vi "GetGlobalDefaultConfiguration.vi"(2 "DO NOT override instruments":bool, 3 "Read defaults?":bool) -> (1 "Configuration File IV":path)   [LabVIEW 2013]
uses:
  QC_MeasurementSetup.vi
  InstrControl/InstrControl.lvclass
panel:
  out "Configuration File Cis":path
  out "Configuration File Stability":path
  out "Configuration File CV":path
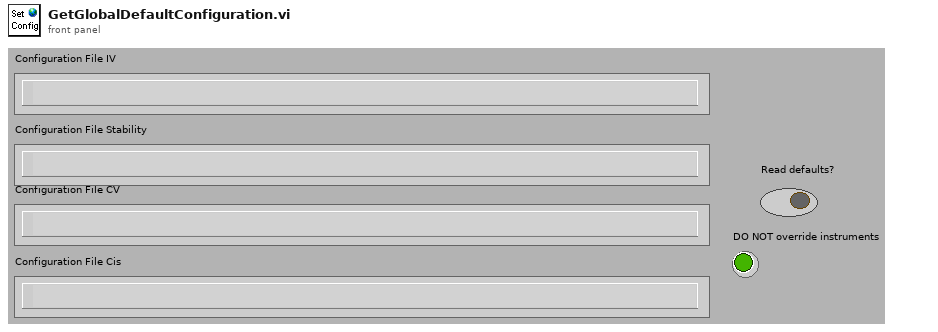
[diagram p1: front panel]
types:
  T1 = cluster{"Supply":refnum<class "SupplyControl.lvclass">, "Initial Voltage [V]":dbl, "Final Voltage [V]":dbl, "Step Size [V]":dbl, "Step Interval [s]":i32, "Number Of Steps":u32, "Ramp down steps [V]":dbl, "Ramp down Interval [s]":i32, "Set Current Limit?":bool, "Current Limit [µA]":dbl, "Temperature Readout":enum16{"Read Arduino", "Enter manually"}, "Arduino":refnum<class "ArduinoControl.lvclass">, "Supply Name":string, "V_breakdown Limit [V]":dbl, "Switching":refnum<class "Switching.lvclass">, "Matrix used?":bool, "Matrix X Channels":cluster{"Bias Supply / SMU LO":i32, "Bias Supply / SMU HI":i32, "CV Box LO":i32, "CV Box HI":i32, "CV Box LO IN":i32, "CV Box HI IN":i32, "Volt meter LO":i32, "Volt meter HI":i32, "Mux1 C1":i32, "Mux1 C2":i32, "Mux2 C1":i32, "Mux2 C2":i32}}
  T2 = cluster{"Supply":refnum<class "SupplyControl.lvclass">, "LCR":refnum<class "LCRControl.lvclass">, "Initial Voltage [V]":dbl, "Final Voltage [V]":dbl, "Step Size [V]":dbl, "Step Interval [s]":i32, "Number Of Steps":u32, "AC frequency [Hz]":i32, "RC Configuration":u16, "AC amplitude [V]":dbl, "Ramp down steps [V]":dbl, "Ramp down Interval [s]":i32, "Set Current Limit?":bool, "Current Limit [µA]":dbl, "Temperature Readout":enum16{"Read Arduino", "Enter manually"}, "Arduino":refnum<class "ArduinoControl.lvclass">, "Supply Name":string, "LCR Name":string, "V_depletion Limit [V]":dbl, "Switching":refnum<class "Switching.lvclass">, "Matrix used?":bool, "Matrix X Channels":cluster{"Bias Supply / SMU LO":i32, "Bias Supply / SMU HI":i32, "CV Box LO":i32, "CV Box HI":i32, "CV Box LO IN":i32, "CV Box HI IN":i32, "Volt meter LO":i32, "Volt meter HI":i32, "Mux1 C1":i32, "Mux1 C2":i32, "Mux2 C1":i32, "Mux2 C2":i32}}
  T3 = cluster{"Supply":refnum<class "SupplyControl.lvclass">, "Voltage [V]":dbl, "Measurement Interval [s]":i32, "Test Duration":u32, "Ramp up steps [V]":dbl, "Ramp up Interval [s]":u32, "Ramp down steps [V]":dbl, "Ramp down Interval [s]":i32, "Set Current Limit?":bool, "Current Limit [µA]":dbl, "Temperature Readout":enum16{"Read Arduino", "Enter manually"}, "Arduino":refnum<class "ArduinoControl.lvclass">, "Supply Name":string, "Maximum current fluctuation [%]":dbl, "Switching.lvclass":refnum<class "Switching.lvclass">, "Matrix used?":bool, "Matrix X Channels":cluster{"Bias Supply / SMU LO":i32, "Bias Supply / SMU HI":i32, "CV Box LO":i32, "CV Box HI":i32, "CV Box LO IN":i32, "CV Box HI IN":i32, "Volt meter LO":i32, "Volt meter HI":i32, "Mux1 C1":i32, "Mux1 C2":i32, "Mux2 C1":i32, "Mux2 C2":i32}}
  T4 = cluster{"Supply":refnum<class "SupplyControl.lvclass">, "LCR":refnum<class "LCRControl.lvclass">, "Initial Voltage [V]":dbl, "Final Voltage [V]":dbl, "Step Size [V]":dbl, "Step Interval [s]":i32, "Number Of Steps":u32, "AC frequency [Hz]":i32, "RC Configuration":u16, "AC amplitude [V]":dbl, "Ramp down steps [V]":dbl, "Ramp down Interval [s]":i32, "Set Current Limit?":bool, "Current Limit [µA]":dbl, "Temperature Readout":enum16{"Read Arduino", "Enter manually"}, "Arduino":refnum<class "ArduinoControl.lvclass">, "Supply Name":string, "LCR Name":string, "C_is Limit [pF/cm]":dbl, "Switching":refnum<class "Switching.lvclass">, "Matrix used?":bool, "Matrix X Channels":cluster{"Bias Supply / SMU LO":i32, "Bias Supply / SMU HI":i32, "CV Box LO":i32, "CV Box HI":i32, "CV Box LO IN":i32, "CV Box HI IN":i32, "Volt meter LO":i32, "Volt meter HI":i32, "Mux1 C1":i32, "Mux1 C2":i32, "Mux2 C1":i32, "Mux2 C2":i32}}
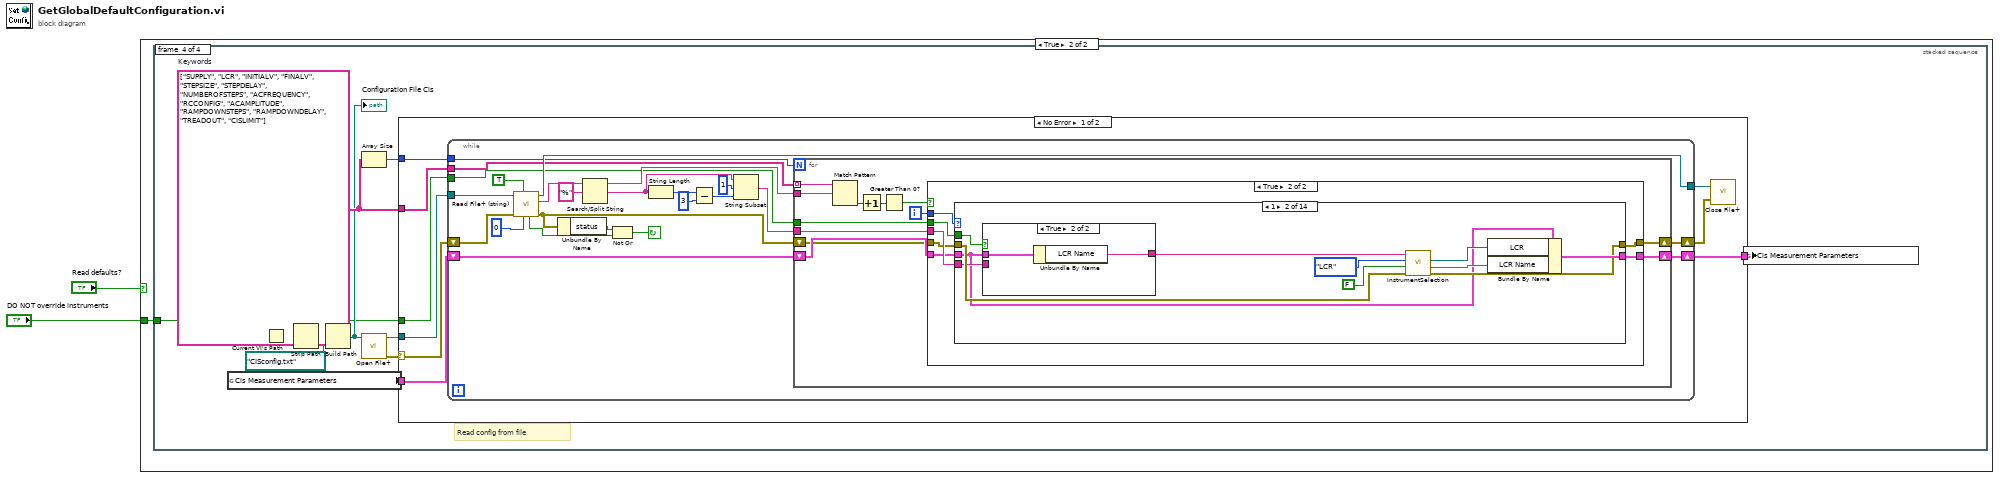
[diagram p0: block diagram]
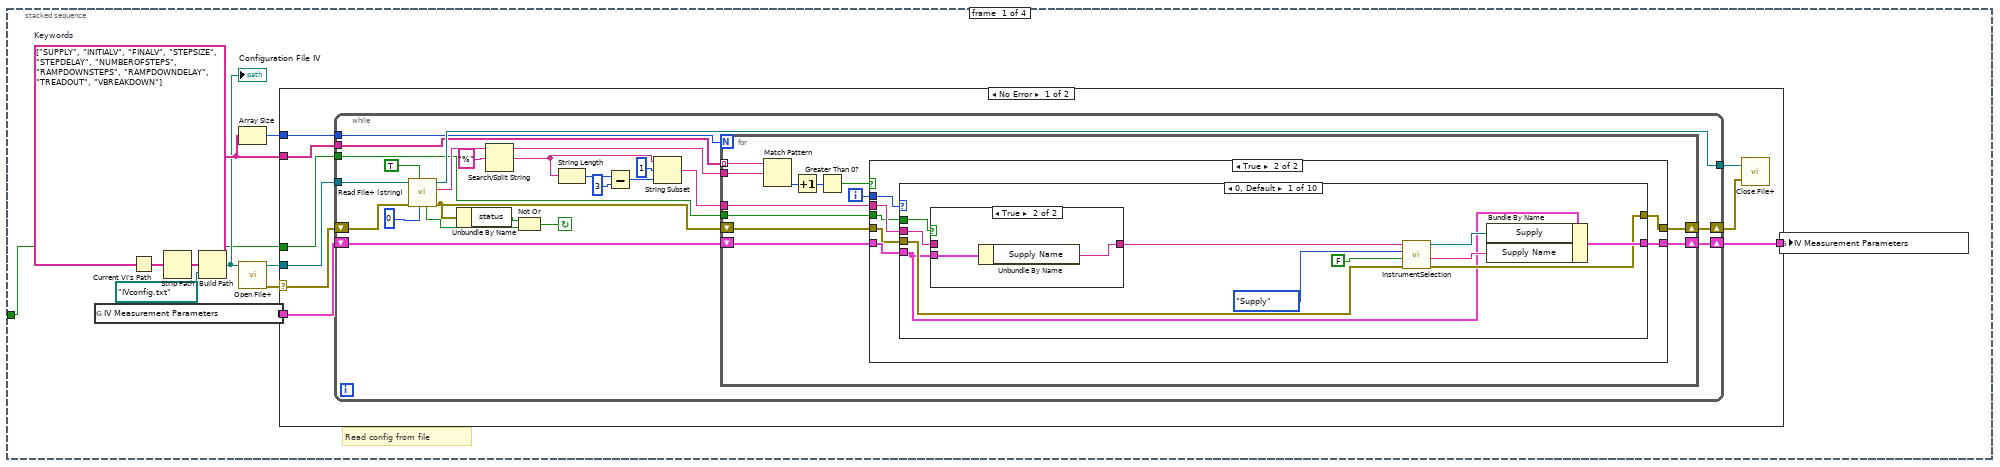
[diagram p3: hidden frame]
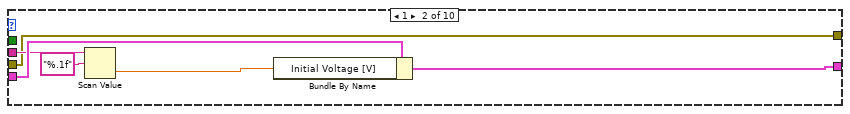
[diagram p6: hidden frame]
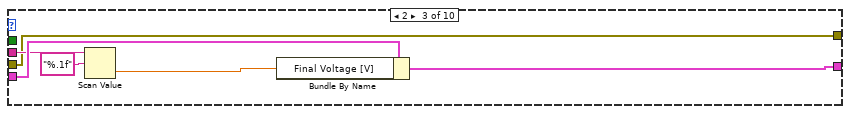
[diagram p7: hidden frame]
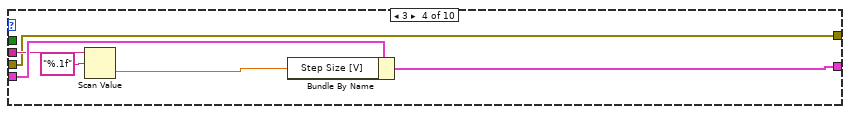
[diagram p8: hidden frame]
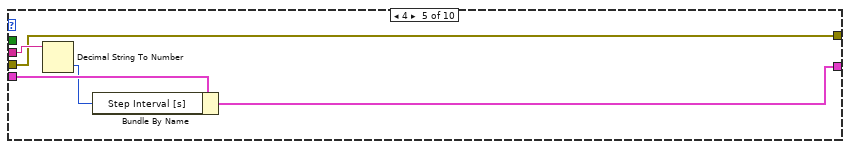
[diagram p9: hidden frame]
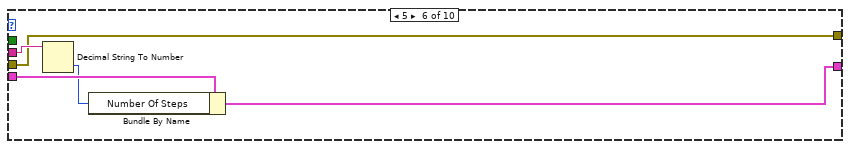
[diagram p10: hidden frame]
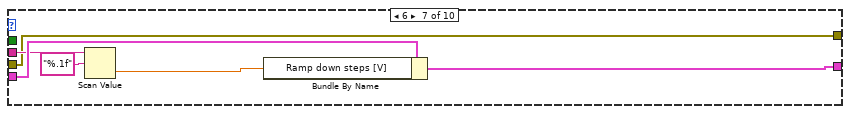
[diagram p11: hidden frame]
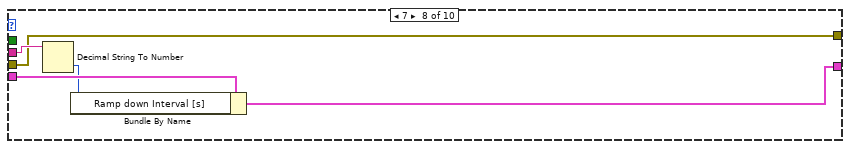
[diagram p12: hidden frame]
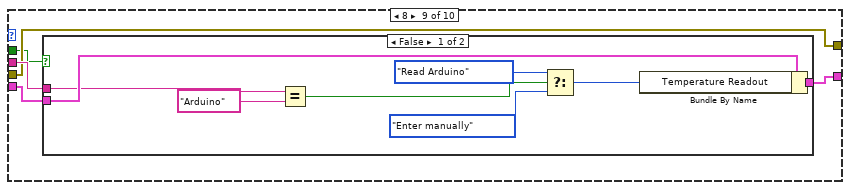
[diagram p13: hidden frame]
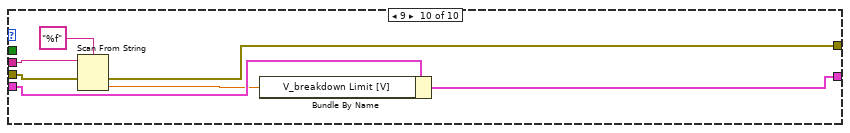
[diagram p15: hidden frame]
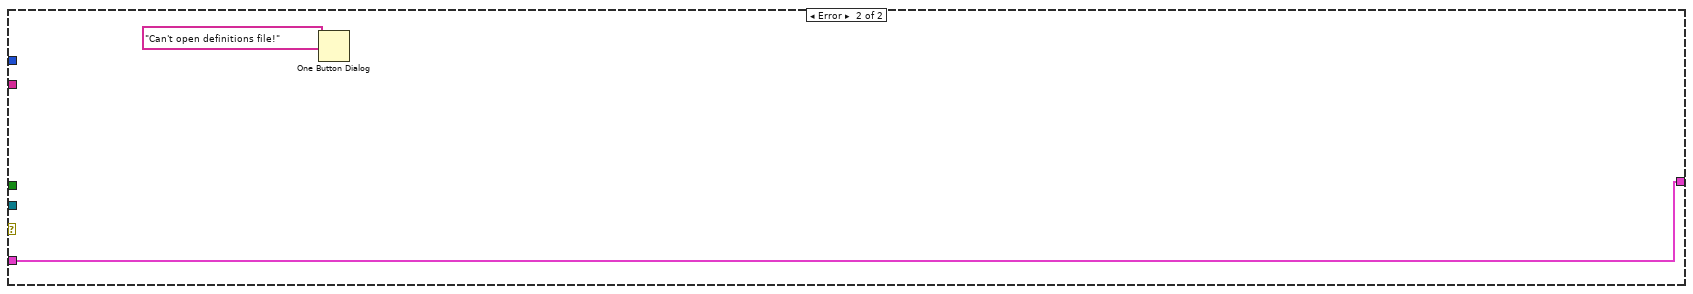
[diagram p16: hidden frame]
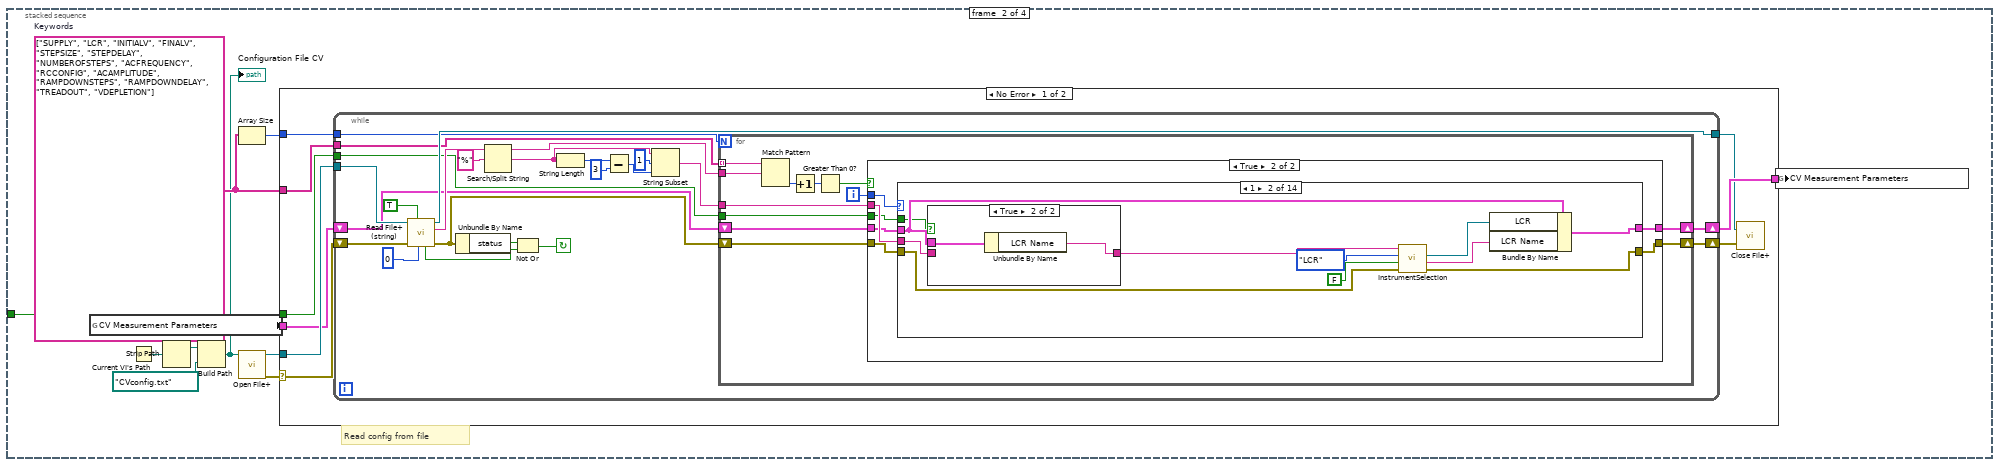
[diagram p17: hidden frame]
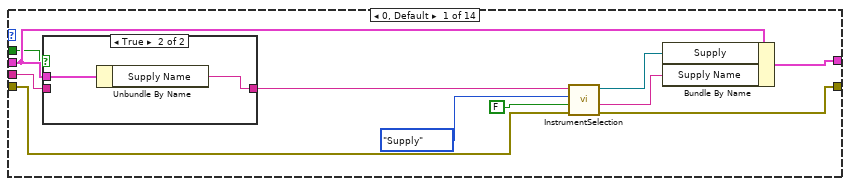
[diagram p19: hidden frame]
diagram:
  n1 = case shown="True" "Read defaults?" {
    tunnel: "DO NOT override instruments" -> [_ w3]
    frame False {
    }
    frame True {
      n2 = stacked-sequence {
        tunnel: w3 -> [w4 w145 w320 w460]
        frame #0 {
          w14 = string[] ["SUPPLY", "INITIALV", "FINALV", "STEPSIZE", "STEPDELAY", "NUMBEROFSTEPS", "RAMPDOWNSTEPS", "RAMPDOWNDELAY", "TREADOUT", "VBREAKDOWN"]  # Keywords
          # "Read config from file"
          n3 = global read "QC_MeasurementSetup.vi" "IV Measurement Parameters"() -> (w5:T1)
          n4 = Current VI's Path() -> (path=w9:path)
          n5 = Strip Path(path=w9) -> (stripped path=w8:path)  [unwired: 1 out]
          n6 = Build Path(base path=w8, name or relative path=path "IVconfig.txt") -> (appended path=w7:path)
          "Configuration File IV" <- w7
          n7 = Array Size(array=w14) -> (size(s)=w13:i32)
          n8 = call <vilib>:"Open File+.vi"("file path (\" \")"=w7) -> ("error out"=w10:errorcluster, "refnum"=w11:refnum<file>)  [unwired: 7 in, 2 out]
          n9 = case shown="No Error" w10 {
            selector: w10 -> [w16 _]
            tunnel: w11 -> [w23 _]
            tunnel: w14 -> [w22 _]
            tunnel: w13 -> [w21 _]
            tunnel: w5 -> [w20 w143]
            tunnel: [w19 w143] -> w6
            tunnel: w4 -> [w15 _]
            frame No Error {
              n10 = while {
                shift-left: w20 -> [w30]
                shift-right: [w28] -> w19
                tunnel: w21 -> [w27]
                tunnel: w22 -> [w33]
                tunnel: [w38] -> w18
                tunnel: w23 -> [w44]
                shift-right: [w25] -> w17
                shift-left: w16 -> [w37]
                tunnel: w15 -> [w24]
                stop <- w40 continue-if-true
                n11 = call <vilib>:"Read File+ (string).vi"("count"=0, "line mode (characters:F)"=TRUE, "error in (no error)"=w37, "refnum"=w44) -> ("error out"=w26:errorcluster, "string"=w39:string, "dup refnum"=w38:refnum<file>, "EOF?"=w42:bool)  [unwired: 3 in, 1 out]
                n12 = Unbundle By Name(w26) -> ("status"=w41:bool)
                n13 = Search/Split String(string=w39, search string/char (-)="%" ("search char (-)")) -> (substring before match=w32:string, match + rest of string=w45:string)  [unwired: 1 in, 1 out]
                n14 = Not Or(1:w42, 2:w41) -> (0:w40:bool)
                n15 = String Length(string=w45) -> (length=w31:i32)
                n16 = Subtract(x=w31, y=3) -> (x-y=w34:i32)
                n17 = String Subset(string=w45, offset (0)=1, length (rest)=w34) -> (substring=w29:string)
                n18 = for {
                  N: w27 -> [_]
                  tunnel: w33 -> [w57] mode=indexing
                  tunnel: w32 -> [w52]
                  shift-right: [w53] -> w28
                  shift-left: w30 -> [w54]
                  tunnel: w29 -> [w51]
                  shift-right: [w49] -> w25
                  shift-left: w26 -> [w50]
                  tunnel: w24 -> [w48]
                  i -> [w55]
                  n19 = Match Pattern(string=w57, regular expression=w52) -> (offset past match=w58:i32)  [unwired: 1 in, 3 out]
                  n20 = Increment(x=w58) -> (x+1=w59:i32)
                  n21 = Greater Than 0?(x=w59) -> (x > 0?=w56:bool)
                  n22 = case shown="True" w56 {
                    tunnel: w55 -> [_ w68]
                    tunnel: w51 -> [_ w67]
                    tunnel: w54 -> [w61 w66]
                    tunnel: [w61 w65] -> w53
                    tunnel: w50 -> [w60 w64]
                    tunnel: [w60 w63] -> w49
                    tunnel: w48 -> [_ w62]
                    frame False {
                    }
                    frame True {
                      n23 = case shown="0, Default" w68 {
                        tunnel: w67 -> [w73 w86 w91 w97 w103 w108 w113 w119 w124 w140]
                        tunnel: w66 -> [w72 w88 w94 w100 w105 w110 w116 w121 w126 w142]
                        tunnel: [w79 w87 w93 w99 w104 w109 w115 w120 w125 w141] -> w65
                        tunnel: w64 -> [w78 w83 w89 w95 w101 w106 w111 w117 w123 w137]
                        tunnel: [w77 w83 w89 w95 w101 w106 w111 w117 w123 w136] -> w63
                        tunnel: w62 -> [w70 _ _ _ _ _ _ _ w122 _]
                        frame 0, Default {
                          n24 = case shown="True" w70 {
                            tunnel: w73 -> [w80 _]
                            tunnel: [w80 w81] -> w71
                            tunnel: w72 -> [_ w82]
                            frame False {
                            }
                            frame True {
                              n25 = Unbundle By Name(w82) -> ("Supply Name"=w81:string)
                            }
                          }
                          n26 = call "InstrumentSelection.vi"("error in (no error)"=w78, "Verify GPIB address"=FALSE, "Instrument type"=enum16{"Supply", "LCR", "Multimeter"}."Supply", "Instrument name IN"=w71) -> ("error out"=w77:errorcluster, "Instrument name OUT"=w76:string, "Supply"=w75:refnum<class "SupplyControl.lvclass">)  [unwired: 2 in, 3 out]
                          n27 = Bundle By Name(cluster=w72, "Supply"=w75, "Supply Name"=w76) -> (w79:T1)
                        }
                        frame 1 {
                          n28 = Scan Value(string=w86, format string="%.1f") -> (value=w85:dbl)  [unwired: 1 in, 1 out]
                          n29 = Bundle By Name(cluster=w88, "Initial Voltage [V]"=w85) -> (w87:T1)
                        }
                        frame 2 {
                          n30 = Scan Value(string=w91, format string="%.1f") -> (value=w90:dbl)  [unwired: 1 in, 1 out]
                          n31 = Bundle By Name(cluster=w94, "Final Voltage [V]"=w90) -> (w93:T1)
                        }
                        frame 3 {
                          n32 = Scan Value(string=w97, format string="%.1f") -> (value=w96:dbl)  [unwired: 1 in, 1 out]
                          n33 = Bundle By Name(cluster=w100, "Step Size [V]"=w96) -> (w99:T1)
                        }
                        frame 4 {
                          n34 = Decimal String To Number(string=w103) -> (number=w102:i32)  [unwired: 2 in, 1 out]
                          n35 = Bundle By Name(cluster=w105, "Step Interval [s]"=w102) -> (w104:T1)
                        }
                        frame 5 {
                          n36 = Decimal String To Number(string=w108) -> (number=w107:i32)  [unwired: 2 in, 1 out]
                          n37 = Bundle By Name(cluster=w110, "Number Of Steps"=w107) -> (w109:T1)
                        }
                        frame 6 {
                          n38 = Scan Value(string=w113, format string="%.1f") -> (value=w112:dbl)  [unwired: 1 in, 1 out]
                          n39 = Bundle By Name(cluster=w116, "Ramp down steps [V]"=w112) -> (w115:T1)
                        }
                        frame 7 {
                          n40 = Decimal String To Number(string=w119) -> (number=w118:i32)  [unwired: 2 in, 1 out]
                          n41 = Bundle By Name(cluster=w121, "Ramp down Interval [s]"=w118) -> (w120:T1)
                        }
                        frame 8 {
                          n42 = case shown="False" w122 {
                            tunnel: w126 -> [w134 w135]
                            tunnel: [w133 w135] -> w125
                            tunnel: w124 -> [w132 _]
                            frame False {
                              n43 = Equal?(x=w132, y="Arduino") -> (x = y?=w130:bool)
                              n44 = Select(t=enum16{"Read Arduino", "Enter manually"}."Read Arduino" ("Temperature Readout"), s=w130, f=enum16{"Read Arduino", "Enter manually"}."Enter manually" ("Temperature Readout")) -> (s? t:f=w127:enum16{"Read Arduino", "Enter manually"})
                              n45 = Bundle By Name(cluster=w134, "Temperature Readout"=w127) -> (w133:T1)
                            }
                            frame True {
                            }
                          }
                        }
                        frame 9 {
                          n46 = Scan From String(format string="%f", input string=w140, error in=w137) -> (error out=w136:errorcluster, output 1=w139:dbl)  [unwired: 2 in, 2 out]
                          n47 = Bundle By Name(cluster=w142, "V_breakdown Limit [V]"=w139) -> (w141:T1)
                        }
                      }
                    }
                  }
                }
              }
              n48 = call <vilib>:"Close File+.vi"("error in (no error)"=w17, "refnum"=w18) -> ()  [unwired: 3 in, 3 out]
            }
            frame Error {
              n49 = One Button Dialog(message="Can't open definitions file!") -> ()  [unwired: 1 in, 1 out]
            }
          }
          n50 = global write "QC_MeasurementSetup.vi" "IV Measurement Parameters"(w6) -> ()
        }
        frame #1 {
          w155 = string[] ["SUPPLY", "LCR", "INITIALV", "FINALV", "STEPSIZE", "STEPDELAY", "NUMBEROFSTEPS", "ACFREQUENCY", "RCCONFIG", "ACAMPLITUDE", "RAMPDOWNSTEPS", "RAMPDOWNDELAY", "TREADOUT", "VDEPLETION"]  # Keywords
          # "Read config from file"
          n51 = global read "QC_MeasurementSetup.vi" "CV Measurement Parameters"() -> (w146:T2)
          n52 = Current VI's Path() -> (path=w150:path)
          n53 = Strip Path(path=w150) -> (stripped path=w149:path)  [unwired: 1 out]
          n54 = Build Path(base path=w149, name or relative path=path "CVconfig.txt") -> (appended path=w148:path)
          "Configuration File CV" <- w148
          n55 = Array Size(array=w155) -> (size(s)=w154:i32)
          n56 = call <vilib>:"Open File+.vi"("file path (\" \")"=w148) -> ("error out"=w151:errorcluster, "refnum"=w152:refnum<file>)  [unwired: 7 in, 2 out]
          n57 = case shown="No Error" w151 {
            selector: w151 -> [w157 _]
            tunnel: w152 -> [w164 _]
            tunnel: w155 -> [w163 _]
            tunnel: w154 -> [w162 _]
            tunnel: w146 -> [w161 w318]
            tunnel: [w160 w318] -> w147
            tunnel: w145 -> [w156 _]
            frame No Error {
              n58 = while {
                shift-left: w161 -> [w171]
                shift-right: [w169] -> w160
                tunnel: w162 -> [w168]
                tunnel: w163 -> [w174]
                tunnel: [w179] -> w159
                tunnel: w164 -> [w185]
                shift-right: [w166] -> w158
                shift-left: w157 -> [w178]
                tunnel: w156 -> [w165]
                stop <- w181 continue-if-true
                n59 = call <vilib>:"Read File+ (string).vi"("count"=0, "line mode (characters:F)"=TRUE, "error in (no error)"=w178, "refnum"=w185) -> ("error out"=w167:errorcluster, "string"=w180:string, "dup refnum"=w179:refnum<file>, "EOF?"=w183:bool)  [unwired: 3 in, 1 out]
                n60 = Unbundle By Name(w167) -> ("status"=w182:bool)
                n61 = Search/Split String(string=w180, search string/char (-)="%" ("search char (-)")) -> (substring before match=w173:string, match + rest of string=w186:string)  [unwired: 1 in, 1 out]
                n62 = Not Or(1:w183, 2:w182) -> (0:w181:bool)
                n63 = String Length(string=w186) -> (length=w172:i32)
                n64 = Subtract(x=w172, y=3) -> (x-y=w175:i32)
                n65 = String Subset(string=w186, offset (0)=1, length (rest)=w175) -> (substring=w170:string)
                n66 = for {
                  N: w168 -> [_]
                  tunnel: w174 -> [w198] mode=indexing
                  tunnel: w173 -> [w193]
                  shift-right: [w194] -> w169
                  shift-left: w171 -> [w195]
                  tunnel: w170 -> [w192]
                  shift-right: [w190] -> w166
                  shift-left: w167 -> [w191]
                  tunnel: w165 -> [w189]
                  i -> [w196]
                  n67 = Match Pattern(string=w198, regular expression=w193) -> (offset past match=w199:i32)  [unwired: 1 in, 3 out]
                  n68 = Increment(x=w199) -> (x+1=w200:i32)
                  n69 = Greater Than 0?(x=w200) -> (x > 0?=w197:bool)
                  n70 = case shown="True" w197 {
                    tunnel: w196 -> [_ w209]
                    tunnel: w192 -> [_ w208]
                    tunnel: w195 -> [w202 w207]
                    tunnel: [w202 w206] -> w194
                    tunnel: w191 -> [w201 w205]
                    tunnel: [w201 w204] -> w190
                    tunnel: w189 -> [_ w203]
                    frame False {
                    }
                    frame True {
                      n71 = case shown="1" w209 {
                        tunnel: w208 -> [w213 w228 w241 w246 w252 w258 w263 w268 w276 w285 w288 w294 w299 w315]
                        tunnel: w207 -> [w214 w227 w243 w249 w255 w260 w265 w270 w279 w283 w291 w296 w301 w311]
                        tunnel: [w220 w234 w242 w248 w254 w259 w264 w269 w278 w281 w290 w295 w300 w312] -> w206
                        tunnel: w205 -> [w218 w233 w238 w244 w250 w256 w261 w266 w271 w280 w286 w292 w298 w314]
                        tunnel: [w219 w232 w238 w244 w250 w256 w261 w266 w271 w280 w286 w292 w298 w313] -> w204
                        tunnel: w203 -> [w211 w225 _ _ _ _ _ _ _ _ _ _ w297 _]
                        frame 0, Default {
                          n72 = case shown="True" w211 {
                            tunnel: w213 -> [w221 _]
                            tunnel: [w221 w222] -> w212
                            tunnel: w214 -> [_ w223]
                            frame False {
                            }
                            frame True {
                              n73 = Unbundle By Name(w223) -> ("Supply Name"=w222:string)
                            }
                          }
                          n74 = call "InstrumentSelection.vi"("error in (no error)"=w218, "Verify GPIB address"=FALSE, "Instrument type"=enum16{"Supply", "LCR", "Multimeter"}."Supply", "Instrument name IN"=w212) -> ("error out"=w219:errorcluster, "Instrument name OUT"=w216:string, "Supply"=w217:refnum<class "SupplyControl.lvclass">)  [unwired: 2 in, 3 out]
                          n75 = Bundle By Name(cluster=w214, "Supply"=w217, "Supply Name"=w216) -> (w220:T2)
                        }
                        frame 1 {
                          n76 = case shown="True" w225 {
                            tunnel: w228 -> [w235 _]
                            tunnel: [w235 w236] -> w226
                            tunnel: w227 -> [_ w237]
                            frame False {
                            }
                            frame True {
                              n77 = Unbundle By Name(w237) -> ("LCR Name"=w236:string)
                            }
                          }
                          n78 = call "InstrumentSelection.vi"("error in (no error)"=w233, "Verify GPIB address"=FALSE, "Instrument type"=enum16{"Supply", "LCR", "Multimeter"}."LCR", "Instrument name IN"=w226) -> ("error out"=w232:errorcluster, "Instrument name OUT"=w231:string, "LCR"=w230:refnum<class "LCRControl.lvclass">)  [unwired: 2 in, 3 out]
                          n79 = Bundle By Name(cluster=w227, "LCR"=w230, "LCR Name"=w231) -> (w234:T2)
                        }
                        frame 2 {
                          n80 = Scan Value(string=w241, format string="%.1f") -> (value=w240:dbl)  [unwired: 1 in, 1 out]
                          n81 = Bundle By Name(cluster=w243, "Initial Voltage [V]"=w240) -> (w242:T2)
                        }
                        frame 3 {
                          n82 = Scan Value(string=w246, format string="%.1f") -> (value=w245:dbl)  [unwired: 1 in, 1 out]
                          n83 = Bundle By Name(cluster=w249, "Final Voltage [V]"=w245) -> (w248:T2)
                        }
                        frame 4 {
                          n84 = Scan Value(string=w252, format string="%.1f") -> (value=w251:dbl)  [unwired: 1 in, 1 out]
                          n85 = Bundle By Name(cluster=w255, "Step Size [V]"=w251) -> (w254:T2)
                        }
                        frame 5 {
                          n86 = Decimal String To Number(string=w258) -> (number=w257:i32)  [unwired: 2 in, 1 out]
                          n87 = Bundle By Name(cluster=w260, "Step Interval [s]"=w257) -> (w259:T2)
                        }
                        frame 6 {
                          n88 = Decimal String To Number(string=w263) -> (number=w262:i32)  [unwired: 2 in, 1 out]
                          n89 = Bundle By Name(cluster=w265, "Number Of Steps"=w262) -> (w264:T2)
                        }
                        frame 7 {
                          n90 = Decimal String To Number(string=w268) -> (number=w267:i32)  [unwired: 2 in, 1 out]
                          n91 = Bundle By Name(cluster=w270, "AC frequency [Hz]"=w267) -> (w269:T2)
                        }
                        frame 8 {
                          w275 = u16 0 items=["serial", "parallel"] ("RC Configuration")
                          w274 = u16 1 items=["serial", "parallel"] ("RC Configuration")
                          n92 = Equal?(x=w276, y="serial") -> (x = y?=w273:bool)
                          n93 = Select(t=w275, s=w273, f=w274) -> (s? t:f=w272:u16)
                          n94 = Bundle By Name(cluster=w279, "RC Configuration"=w272) -> (w278:T2)
                        }
                        frame 9 {
                          n95 = Scan Value(string=w285, format string="%.1f") -> (value=w282:dbl)  [unwired: 1 in, 1 out]
                          n96 = Bundle By Name(cluster=w283, "AC amplitude [V]"=w282) -> (w281:T2)
                        }
                        frame 10 {
                          n97 = Scan Value(string=w288, format string="%.1f") -> (value=w287:dbl)  [unwired: 1 in, 1 out]
                          n98 = Bundle By Name(cluster=w291, "Ramp down steps [V]"=w287) -> (w290:T2)
                        }
                        frame 11 {
                          n99 = Decimal String To Number(string=w294) -> (number=w293:i32)  [unwired: 2 in, 1 out]
                          n100 = Bundle By Name(cluster=w296, "Ramp down Interval [s]"=w293) -> (w295:T2)
                        }
                        frame 12 {
                          n101 = case shown="False" w297 {
                            tunnel: w301 -> [w309 w310]
                            tunnel: [w308 w310] -> w300
                            tunnel: w299 -> [w307 _]
                            frame False {
                              n102 = Equal?(x=w307, y="Arduino") -> (x = y?=w305:bool)
                              n103 = Select(t=enum16{"Read Arduino", "Enter manually"}."Read Arduino" ("Temperature Readout"), s=w305, f=enum16{"Read Arduino", "Enter manually"}."Enter manually" ("Temperature Readout")) -> (s? t:f=w302:enum16{"Read Arduino", "Enter manually"})
                              n104 = Bundle By Name(cluster=w309, "Temperature Readout"=w302) -> (w308:T2)
                            }
                            frame True {
                            }
                          }
                        }
                        frame 13 {
                          n105 = Scan From String(format string="%f", input string=w315, error in=w314) -> (error out=w313:errorcluster, output 1=w317:dbl)  [unwired: 2 in, 2 out]
                          n106 = Bundle By Name(cluster=w311, "V_depletion Limit [V]"=w317) -> (w312:T2)
                        }
                      }
                    }
                  }
                }
              }
              n107 = call <vilib>:"Close File+.vi"("error in (no error)"=w158, "refnum"=w159) -> ()  [unwired: 3 in, 3 out]
            }
            frame Error {
              n108 = One Button Dialog(message="Can't open definitions file!") -> ()  [unwired: 1 in, 1 out]
            }
          }
          n109 = global write "QC_MeasurementSetup.vi" "CV Measurement Parameters"(w147) -> ()
        }
        frame #2 {
          w330 = string[] ["SUPPLY", "VOLTAGE", "INTERVAL", "DURATION", "RAMPUPSTEPS", "RAMPUPDELAY", "RAMPDOWNSTEPS", "RAMPDOWNDELAY", "TREADOUT", "IFLUCTUATIONS"]  # Keywords
          # "Read config from file"
          n110 = global read "QC_MeasurementSetup.vi" "Current Stability Measurement Parameters"() -> (w321:T3)
          n111 = Current VI's Path() -> (path=w325:path)
          n112 = Strip Path(path=w325) -> (stripped path=w324:path)  [unwired: 1 out]
          n113 = Build Path(base path=w324, name or relative path=path "STABILITYconfig.txt") -> (appended path=w323:path)
          "Configuration File Stability" <- w323
          n114 = Array Size(array=w330) -> (size(s)=w329:i32)
          n115 = call <vilib>:"Open File+.vi"("file path (\" \")"=w323) -> ("error out"=w326:errorcluster, "refnum"=w327:refnum<file>)  [unwired: 7 in, 2 out]
          n116 = case shown="No Error" w326 {
            selector: w326 -> [w332 _]
            tunnel: w327 -> [w339 _]
            tunnel: w330 -> [w338 _]
            tunnel: w329 -> [w337 _]
            tunnel: w321 -> [w336 w458]
            tunnel: [w335 w458] -> w322
            tunnel: w320 -> [w331 _]
            frame No Error {
              n117 = while {
                shift-left: w336 -> [w346]
                shift-right: [w344] -> w335
                tunnel: w337 -> [w343]
                tunnel: w338 -> [w349]
                tunnel: [w354] -> w334
                tunnel: w339 -> [w360]
                shift-right: [w341] -> w333
                shift-left: w332 -> [w353]
                tunnel: w331 -> [w340]
                stop <- w356 continue-if-true
                n118 = call <vilib>:"Read File+ (string).vi"("count"=0, "line mode (characters:F)"=TRUE, "error in (no error)"=w353, "refnum"=w360) -> ("error out"=w342:errorcluster, "string"=w355:string, "dup refnum"=w354:refnum<file>, "EOF?"=w358:bool)  [unwired: 3 in, 1 out]
                n119 = Unbundle By Name(w342) -> ("status"=w357:bool)
                n120 = Search/Split String(string=w355, search string/char (-)="%" ("search char (-)")) -> (substring before match=w348:string, match + rest of string=w361:string)  [unwired: 1 in, 1 out]
                n121 = Not Or(1:w358, 2:w357) -> (0:w356:bool)
                n122 = String Length(string=w361) -> (length=w347:i32)
                n123 = Subtract(x=w347, y=3) -> (x-y=w350:i32)
                n124 = String Subset(string=w361, offset (0)=1, length (rest)=w350) -> (substring=w345:string)
                n125 = for {
                  N: w343 -> [_]
                  tunnel: w349 -> [w373] mode=indexing
                  tunnel: w348 -> [w368]
                  shift-right: [w369] -> w344
                  shift-left: w346 -> [w370]
                  tunnel: w345 -> [w367]
                  shift-right: [w365] -> w341
                  shift-left: w342 -> [w366]
                  tunnel: w340 -> [w364]
                  i -> [w371]
                  n126 = Match Pattern(string=w373, regular expression=w368) -> (offset past match=w374:i32)  [unwired: 1 in, 3 out]
                  n127 = Increment(x=w374) -> (x+1=w375:i32)
                  n128 = Greater Than 0?(x=w375) -> (x > 0?=w372:bool)
                  n129 = case shown="True" w372 {
                    tunnel: w371 -> [_ w384]
                    tunnel: w367 -> [_ w383]
                    tunnel: w370 -> [w377 w382]
                    tunnel: [w377 w381] -> w369
                    tunnel: w366 -> [w376 w380]
                    tunnel: [w376 w379] -> w365
                    tunnel: w364 -> [_ w378]
                    frame False {
                    }
                    frame True {
                      n130 = case shown="0, Default" w384 {
                        tunnel: w383 -> [w389 w402 w406 w411 w417 w423 w428 w434 w439 w454]
                        tunnel: w382 -> [w386 w404 w409 w414 w420 w425 w431 w436 w441 w455]
                        tunnel: [w395 w403 w408 w413 w419 w424 w430 w435 w440 w453] -> w381
                        tunnel: w380 -> [w394 w399 w407 w412 w418 w421 w426 w432 w438 w451]
                        tunnel: [w393 w399 w407 w412 w418 w421 w426 w432 w438 w452] -> w379
                        tunnel: w378 -> [w387 _ _ _ _ _ _ _ w437 _]
                        frame 0, Default {
                          n131 = case shown="True" w387 {
                            tunnel: w389 -> [w396 _]
                            tunnel: [w396 w397] -> w388
                            tunnel: w386 -> [_ w398]
                            frame False {
                            }
                            frame True {
                              n132 = Unbundle By Name(w398) -> ("Supply Name"=w397:string)
                            }
                          }
                          n133 = call "InstrumentSelection.vi"("error in (no error)"=w394, "Verify GPIB address"=FALSE, "Instrument type"=enum16{"Supply", "LCR", "Multimeter"}."Supply", "Instrument name IN"=w388) -> ("error out"=w393:errorcluster, "Instrument name OUT"=w392:string, "Supply"=w391:refnum<class "SupplyControl.lvclass">)  [unwired: 2 in, 3 out]
                          n134 = Bundle By Name(cluster=w386, "Supply"=w391, "Supply Name"=w392) -> (w395:T3)
                        }
                        frame 1 {
                          n135 = Scan Value(string=w402, format string="%.1f") -> (value=w401:dbl)  [unwired: 1 in, 1 out]
                          n136 = Bundle By Name(cluster=w404, "Voltage [V]"=w401) -> (w403:T3)
                        }
                        frame 2 {
                          n137 = Decimal String To Number(string=w406) -> (number=w405:i32)  [unwired: 2 in, 1 out]
                          n138 = Bundle By Name(cluster=w409, "Measurement Interval [s]"=w405) -> (w408:T3)
                        }
                        frame 3 {
                          n139 = Decimal String To Number(string=w411) -> (number=w410:i32)  [unwired: 2 in, 1 out]
                          n140 = Bundle By Name(cluster=w414, "Test Duration"=w410) -> (w413:T3)
                        }
                        frame 4 {
                          n141 = Scan Value(string=w417, format string="%.1f") -> (value=w415:dbl)  [unwired: 1 in, 1 out]
                          n142 = Bundle By Name(cluster=w420, "Ramp up steps [V]"=w415) -> (w419:T3)
                        }
                        frame 5 {
                          n143 = Decimal String To Number(string=w423) -> (number=w422:i32)  [unwired: 2 in, 1 out]
                          n144 = Bundle By Name(cluster=w425, "Ramp up Interval [s]"=w422) -> (w424:T3)
                        }
                        frame 6 {
                          n145 = Scan Value(string=w428, format string="%.1f") -> (value=w427:dbl)  [unwired: 1 in, 1 out]
                          n146 = Bundle By Name(cluster=w431, "Ramp down steps [V]"=w427) -> (w430:T3)
                        }
                        frame 7 {
                          n147 = Decimal String To Number(string=w434) -> (number=w433:i32)  [unwired: 2 in, 1 out]
                          n148 = Bundle By Name(cluster=w436, "Ramp down Interval [s]"=w433) -> (w435:T3)
                        }
                        frame 8 {
                          n149 = case shown="False" w437 {
                            tunnel: w441 -> [w449 w450]
                            tunnel: [w448 w450] -> w440
                            tunnel: w439 -> [w447 _]
                            frame False {
                              n150 = Equal?(x=w447, y="Arduino") -> (x = y?=w445:bool)
                              n151 = Select(t=enum16{"Read Arduino", "Enter manually"}."Read Arduino" ("Temperature Readout"), s=w445, f=enum16{"Read Arduino", "Enter manually"}."Enter manually" ("Temperature Readout")) -> (s? t:f=w442:enum16{"Read Arduino", "Enter manually"})
                              n152 = Bundle By Name(cluster=w449, "Temperature Readout"=w442) -> (w448:T3)
                            }
                            frame True {
                            }
                          }
                        }
                        frame 9 {
                          n153 = Scan From String(format string="%f", input string=w454, error in=w451) -> (error out=w452:errorcluster, output 1=w457:dbl)  [unwired: 2 in, 2 out]
                          n154 = Bundle By Name(cluster=w455, "Maximum current fluctuation [%]"=w457) -> (w453:T3)
                        }
                      }
                    }
                  }
                }
              }
              n155 = call <vilib>:"Close File+.vi"("error in (no error)"=w333, "refnum"=w334) -> ()  [unwired: 3 in, 3 out]
            }
            frame Error {
              n156 = One Button Dialog(message="Can't open definitions file!") -> ()  [unwired: 1 in, 1 out]
            }
          }
          n157 = global write "QC_MeasurementSetup.vi" "Current Stability Measurement Parameters"(w322) -> ()
        }
        frame #3 {
          w470 = string[] ["SUPPLY", "LCR", "INITIALV", "FINALV", "STEPSIZE", "STEPDELAY", "NUMBEROFSTEPS", "ACFREQUENCY", "RCCONFIG", "ACAMPLITUDE", "RAMPDOWNSTEPS", "RAMPDOWNDELAY", "TREADOUT", "CISLIMIT"]  # Keywords
          # "Read config from file"
          n158 = global read "QC_MeasurementSetup.vi" "Cis Measurement Parameters"() -> (w461:T4)
          n159 = Current VI's Path() -> (path=w465:path)
          n160 = Strip Path(path=w465) -> (stripped path=w464:path)  [unwired: 1 out]
          n161 = Build Path(base path=w464, name or relative path=path "CISconfig.txt") -> (appended path=w463:path)
          "Configuration File Cis" <- w463
          n162 = Array Size(array=w470) -> (size(s)=w469:i32)
          n163 = call <vilib>:"Open File+.vi"("file path (\" \")"=w463) -> ("error out"=w466:errorcluster, "refnum"=w467:refnum<file>)  [unwired: 7 in, 2 out]
          n164 = case shown="No Error" w466 {
            selector: w466 -> [w472 _]
            tunnel: w467 -> [w479 _]
            tunnel: w470 -> [w478 _]
            tunnel: w469 -> [w477 _]
            tunnel: w461 -> [w476 w633]
            tunnel: [w475 w633] -> w462
            tunnel: w460 -> [w471 _]
            frame No Error {
              n165 = while {
                shift-left: w476 -> [w486]
                shift-right: [w484] -> w475
                tunnel: w477 -> [w483]
                tunnel: w478 -> [w489]
                tunnel: [w494] -> w474
                tunnel: w479 -> [w500]
                shift-right: [w481] -> w473
                shift-left: w472 -> [w493]
                tunnel: w471 -> [w480]
                stop <- w496 continue-if-true
                n166 = call <vilib>:"Read File+ (string).vi"("count"=0, "line mode (characters:F)"=TRUE, "error in (no error)"=w493, "refnum"=w500) -> ("error out"=w482:errorcluster, "string"=w495:string, "dup refnum"=w494:refnum<file>, "EOF?"=w498:bool)  [unwired: 3 in, 1 out]
                n167 = Unbundle By Name(w482) -> ("status"=w497:bool)
                n168 = Search/Split String(string=w495, search string/char (-)="%" ("search char (-)")) -> (substring before match=w488:string, match + rest of string=w501:string)  [unwired: 1 in, 1 out]
                n169 = Not Or(1:w498, 2:w497) -> (0:w496:bool)
                n170 = String Length(string=w501) -> (length=w487:i32)
                n171 = Subtract(x=w487, y=3) -> (x-y=w490:i32)
                n172 = String Subset(string=w501, offset (0)=1, length (rest)=w490) -> (substring=w485:string)
                n173 = for {
                  N: w483 -> [_]
                  tunnel: w489 -> [w513] mode=indexing
                  tunnel: w488 -> [w508]
                  shift-right: [w509] -> w484
                  shift-left: w486 -> [w510]
                  tunnel: w485 -> [w507]
                  shift-right: [w505] -> w481
                  shift-left: w482 -> [w506]
                  tunnel: w480 -> [w504]
                  i -> [w511]
                  n174 = Match Pattern(string=w513, regular expression=w508) -> (offset past match=w514:i32)  [unwired: 1 in, 3 out]
                  n175 = Increment(x=w514) -> (x+1=w515:i32)
                  n176 = Greater Than 0?(x=w515) -> (x > 0?=w512:bool)
                  n177 = case shown="True" w512 {
                    tunnel: w511 -> [_ w524]
                    tunnel: w507 -> [_ w523]
                    tunnel: w510 -> [w517 w522]
                    tunnel: [w517 w521] -> w509
                    tunnel: w506 -> [w516 w520]
                    tunnel: [w516 w519] -> w505
                    tunnel: w504 -> [_ w518]
                    frame False {
                    }
                    frame True {
                      n178 = case shown="1" w524 {
                        tunnel: w523 -> [w529 w543 w556 w561 w567 w573 w578 w583 w591 w600 w603 w609 w614 w630]
                        tunnel: w522 -> [w527 w542 w558 w564 w570 w575 w580 w585 w594 w598 w606 w611 w616 w629]
                        tunnel: [w535 w549 w557 w563 w569 w574 w579 w584 w593 w596 w605 w610 w615 w628] -> w521
                        tunnel: w520 -> [w533 w548 w553 w559 w565 w571 w576 w581 w586 w595 w601 w607 w613 w626]
                        tunnel: [w534 w547 w553 w559 w565 w571 w576 w581 w586 w595 w601 w607 w613 w627] -> w519
                        tunnel: w518 -> [w526 w540 _ _ _ _ _ _ _ _ _ _ w612 _]
                        frame 0, Default {
                          n179 = case shown="True" w526 {
                            tunnel: w529 -> [w536 _]
                            tunnel: [w536 w537] -> w528
                            tunnel: w527 -> [_ w538]
                            frame False {
                            }
                            frame True {
                              n180 = Unbundle By Name(w538) -> ("Supply Name"=w537:string)
                            }
                          }
                          n181 = call "InstrumentSelection.vi"("error in (no error)"=w533, "Verify GPIB address"=FALSE, "Instrument type"=enum16{"Supply", "LCR", "Multimeter"}."Supply", "Instrument name IN"=w528) -> ("error out"=w534:errorcluster, "Instrument name OUT"=w531:string, "Supply"=w532:refnum<class "SupplyControl.lvclass">)  [unwired: 2 in, 3 out]
                          n182 = Bundle By Name(cluster=w527, "Supply"=w532, "Supply Name"=w531) -> (w535:T4)
                        }
                        frame 1 {
                          n183 = case shown="True" w540 {
                            tunnel: w543 -> [w550 _]
                            tunnel: [w550 w551] -> w541
                            tunnel: w542 -> [_ w552]
                            frame False {
                            }
                            frame True {
                              n184 = Unbundle By Name(w552) -> ("LCR Name"=w551:string)
                            }
                          }
                          n185 = call "InstrumentSelection.vi"("error in (no error)"=w548, "Verify GPIB address"=FALSE, "Instrument type"=enum16{"Supply", "LCR", "Multimeter"}."LCR", "Instrument name IN"=w541) -> ("error out"=w547:errorcluster, "Instrument name OUT"=w546:string, "LCR"=w545:refnum<class "LCRControl.lvclass">)  [unwired: 2 in, 3 out]
                          n186 = Bundle By Name(cluster=w542, "LCR"=w545, "LCR Name"=w546) -> (w549:T4)
                        }
                        frame 2 {
                          n187 = Scan Value(string=w556, format string="%.1f") -> (value=w555:dbl)  [unwired: 1 in, 1 out]
                          n188 = Bundle By Name(cluster=w558, "Initial Voltage [V]"=w555) -> (w557:T4)
                        }
                        frame 3 {
                          n189 = Scan Value(string=w561, format string="%.1f") -> (value=w560:dbl)  [unwired: 1 in, 1 out]
                          n190 = Bundle By Name(cluster=w564, "Final Voltage [V]"=w560) -> (w563:T4)
                        }
                        frame 4 {
                          n191 = Scan Value(string=w567, format string="%.1f") -> (value=w566:dbl)  [unwired: 1 in, 1 out]
                          n192 = Bundle By Name(cluster=w570, "Step Size [V]"=w566) -> (w569:T4)
                        }
                        frame 5 {
                          n193 = Decimal String To Number(string=w573) -> (number=w572:i32)  [unwired: 2 in, 1 out]
                          n194 = Bundle By Name(cluster=w575, "Step Interval [s]"=w572) -> (w574:T4)
                        }
                        frame 6 {
                          n195 = Decimal String To Number(string=w578) -> (number=w577:i32)  [unwired: 2 in, 1 out]
                          n196 = Bundle By Name(cluster=w580, "Number Of Steps"=w577) -> (w579:T4)
                        }
                        frame 7 {
                          n197 = Decimal String To Number(string=w583) -> (number=w582:i32)  [unwired: 2 in, 1 out]
                          n198 = Bundle By Name(cluster=w585, "AC frequency [Hz]"=w582) -> (w584:T4)
                        }
                        frame 8 {
                          w590 = u16 0 items=["serial", "parallel"] ("RC Configuration")
                          w589 = u16 1 items=["serial", "parallel"] ("RC Configuration")
                          n199 = Equal?(x=w591, y="serial") -> (x = y?=w588:bool)
                          n200 = Select(t=w590, s=w588, f=w589) -> (s? t:f=w587:u16)
                          n201 = Bundle By Name(cluster=w594, "RC Configuration"=w587) -> (w593:T4)
                        }
                        frame 9 {
                          n202 = Scan Value(string=w600, format string="%.1f") -> (value=w597:dbl)  [unwired: 1 in, 1 out]
                          n203 = Bundle By Name(cluster=w598, "AC amplitude [V]"=w597) -> (w596:T4)
                        }
                        frame 10 {
                          n204 = Scan Value(string=w603, format string="%.1f") -> (value=w602:dbl)  [unwired: 1 in, 1 out]
                          n205 = Bundle By Name(cluster=w606, "Ramp down steps [V]"=w602) -> (w605:T4)
                        }
                        frame 11 {
                          n206 = Decimal String To Number(string=w609) -> (number=w608:i32)  [unwired: 2 in, 1 out]
                          n207 = Bundle By Name(cluster=w611, "Ramp down Interval [s]"=w608) -> (w610:T4)
                        }
                        frame 12 {
                          n208 = case shown="False" w612 {
                            tunnel: w616 -> [w624 w625]
                            tunnel: [w623 w625] -> w615
                            tunnel: w614 -> [w622 _]
                            frame False {
                              n209 = Equal?(x=w622, y="Arduino") -> (x = y?=w620:bool)
                              n210 = Select(t=enum16{"Read Arduino", "Enter manually"}."Read Arduino" ("Temperature Readout"), s=w620, f=enum16{"Read Arduino", "Enter manually"}."Enter manually" ("Temperature Readout")) -> (s? t:f=w617:enum16{"Read Arduino", "Enter manually"})
                              n211 = Bundle By Name(cluster=w624, "Temperature Readout"=w617) -> (w623:T4)
                            }
                            frame True {
                            }
                          }
                        }
                        frame 13 {
                          n212 = Scan From String(format string="%f", input string=w630, error in=w626) -> (error out=w627:errorcluster, output 1=w632:dbl)  [unwired: 2 in, 2 out]
                          n213 = Bundle By Name(cluster=w629, "C_is Limit [pF/cm]"=w632) -> (w628:T4)
                        }
                      }
                    }
                  }
                }
              }
              n214 = call <vilib>:"Close File+.vi"("error in (no error)"=w473, "refnum"=w474) -> ()  [unwired: 3 in, 3 out]
            }
            frame Error {
              n215 = One Button Dialog(message="Can't open definitions file!") -> ()  [unwired: 1 in, 1 out]
            }
          }
          n216 = global write "QC_MeasurementSetup.vi" "Cis Measurement Parameters"(w462) -> ()
        }
      }
    }
  }
